vi "Window-8-bit Export output setup.vi"() -> ()   [LabVIEW 2017]
uses:
  Typedefs/Image selector control.ctl
  Functional Imaging Viewer/Typedefs/Get-Set-Clear Control.ctl
  Typedefs/Image stitching positions.ctl
  Global Variables/General Globals.vi
  Globals/gl_Time series viewer globals.vi
panel:
  in  "Bottom right":T1=enum."\n\nNone"
  in  "Bottom left":T1=enum."\n\nNone"
  in  "Top right":T1=enum."\n\nVideo 1"
  in  "Top left":T1=enum."\n\nNone"
  out "Speed graph":string
  in  "Cancel":bool
  in  "OK":bool
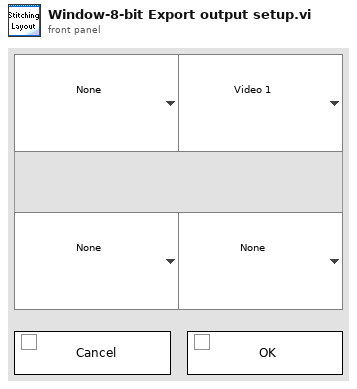
[diagram p1: front panel]
types:
  T1 = typedef "Image selector control.ctl" = enum16{"\n\nTimelapse", "\n\nVideo 1", "\n\nVideo 2", "\n\nVideo 3", "\n\nVideo 4", "\n\nNone"}
  T2 = typedef "Image stitching positions.ctl" = enum16{"Top left", "Top right", "Bottom left", "Bottom right", "Not used"}
  T3 = typedef "Get-Set-Clear Control.ctl" = enum16{"Get", "Set", "Clear"}
  T4 = typedef "Stitch layout spec cluster.ctl" = cluster{"Timelapse image":cluster{"Image position":T2}, "Cam 1":cluster{"Image position":T2}, "Cam 2":cluster{"Image position":T2}, "Cam 3":cluster{"Image position":T2}, "Cam 4":cluster{"Image position":T2}}
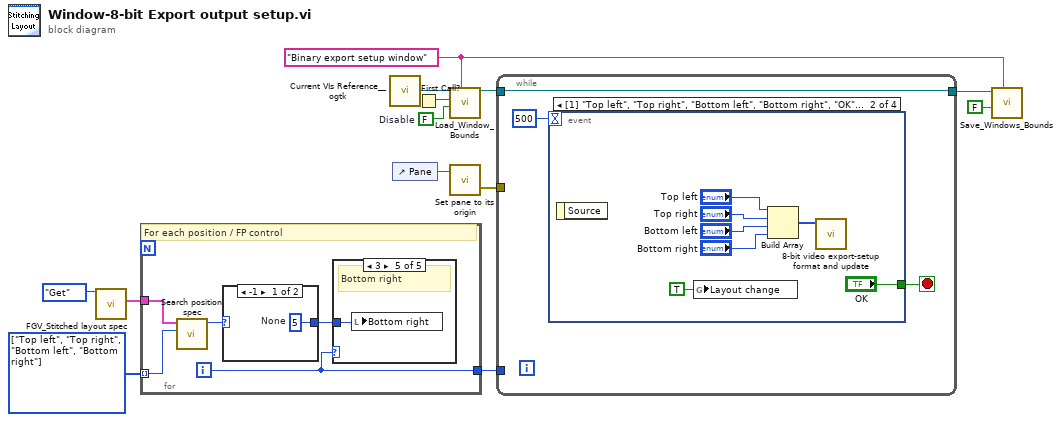
[diagram p0: block diagram]
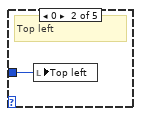
[diagram p4: hidden frame]
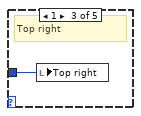
[diagram p5: hidden frame]
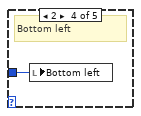
[diagram p6: hidden frame]
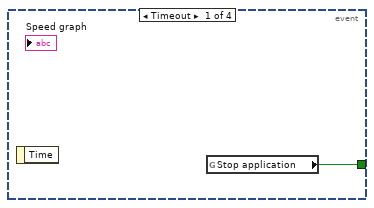
[diagram p7: hidden frame]
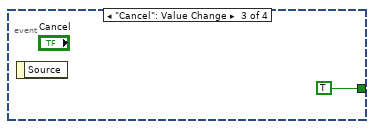
[diagram p8: hidden frame]
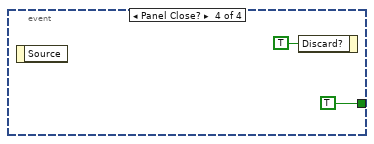
[diagram p9: hidden frame]
diagram:
  w3 = T2[] [enum."Top left", enum."Top right", enum."Bottom left", enum."Bottom right"] items=["Top left", "Top right", "Bottom left", "Bottom right", "Not used"]
  w9 = FALSE  # Disable
  w8 = "Binary export setup window" ("Window Name (i.e. Key)")
  n1 = call "FGV_Stitched layout spec.vi"("Function"=Get-Set-Clear_Control."Get") -> ("Stitch layout spec"=w1:T4)  [unwired: 9 in, 1 out]
  n2 = for {
    tunnel: w1 -> [w18]
    tunnel: w3 -> [w17] mode=indexing
    tunnel: [w14] -> w2
    i -> [w14]
    # "For each position / FP control"
    n3 = call "Search position spec.vi"("Image position"=w17, "Stitch layout spec"=w18) -> ("index of element"=w16:i32)  [unwired: 9 in]
    n4 = case shown="-1" w16 {
      selector: w16 -> [_ w20]
      tunnel: [w19 w20] -> w15
      frame -1 {
        w19 = 5  # None
      }
      frame Default {
      }
    }
    n5 = case shown="3" w14 {
      tunnel: w15 -> [_ w21 w22 w23 w24]
      frame Default {
      }
      frame 0 {
        # "Top left"
        n6 = local write "Top left"(w21) -> ()
      }
      frame 1 {
        # "Top right"
        n7 = local write "Top right"(w22) -> ()
      }
      frame 2 {
        # "Bottom left"
        n8 = local write "Bottom left"(w23) -> ()
      }
      frame 3 {
        # "Bottom right"
        n9 = local write "Bottom right"(w24) -> ()
      }
    }
  }
  n10 = call <userlib>:"Current VIs Reference__ogtk.vi"() -> ("Current VI's reference"=w11:refnum<vi>)  [unwired: 5 in]
  n11 = control-ref of="Pane"() -> (w13:refnum<vi>)
  n12 = First Call?() -> (First Call?: T/F=w10:bool)
  n13 = call "Load_Window_Bounds.vi"("Window Name (i.e. Key)"=w8, "Disable"=w9, "First Call"=w10, "Window VI's Ref"=w11) -> ("reference out"=w5:refnum<vi>)  [unwired: 4 in, 3 out]
  n14 = call <userlib>:"Set pane to its origin.vi"("Pane Reference"=w13) -> ("error out (no error)"=w12:errorcluster)  [unwired: 9 in, 1 out]
  n15 = while {
    tunnel: w12 -> [_]
    tunnel: w5 -> [w27]
    tunnel: [w27] -> w6
    tunnel: w2 -> [_]
    stop <- w25 stop-if-true
    n16 = event shown="[1] \"Top left\", \"Top right\", \"Bottom left\", \"Bottom right\", \"OK\": Value Change" {
      selector: _ -> [_ _ _ _]
      dyn-events: _ -> [_ _ _ _]
      timeout: 500 -> [_ _ _ _]
      tunnel: [w28 "OK" TRUE TRUE] -> w25
      event Timeout {
        n17 = event-data() -> ()  [unwired: 1 in, 1 out]
        n18 = global read "General Globals.vi" "Stop application"() -> (w28:bool)
      }
      event "OK": Value Change {
        n19 = event-data() -> ()  [unwired: 1 in, 1 out]
        n20 = global write "gl_Time series viewer globals.vi" "Layout change"(TRUE ("Layout change")) -> ()
        n21 = Build Array("Top left", "Top right", "Bottom left", "Bottom right") -> (w31:T1[])
        n22 = call "8-bit video export-setup format and update.vi"("Array"=w31) -> ()  [unwired: 11 in]
      }
      event "Cancel": Value Change {
        n23 = event-data() -> ()  [unwired: 1 in, 1 out]
      }
      event Panel Close? {
        n24 = event-data() -> ()  [unwired: 1 in, 1 out]
        n25 = event-data("Discard?"=TRUE) -> ()  [unwired: 1 in, 1 out]
      }
    }
  }
  n26 = call "Save_Windows_Bounds.vi"("Window Name (i.e. Key)"=w8, "Front Panel Window:Open"=FALSE, "Window VI's Ref"=w6) -> ()  [unwired: 8 in, 1 out]
